vi "SaveVIlocations.vi"(10 "NamesAndLocnsArray":T1[](array[typedef]), 11 "configuration file path":path) -> ()   [LabVIEW 2020]
uses:
  <vilib>/Utility/miscctls.llb/LVRectTypeDef.ctl
  <vilib>/Utility/config.llb/Write Key (I32).vi
  <vilib>/Utility/config.llb/NI_LVConfig.lvlib
  <vilib>/Utility/config.llb/Write Key (Path).vi
  Anemometry Sub Vis/Controls/VInameSizePath.ctl
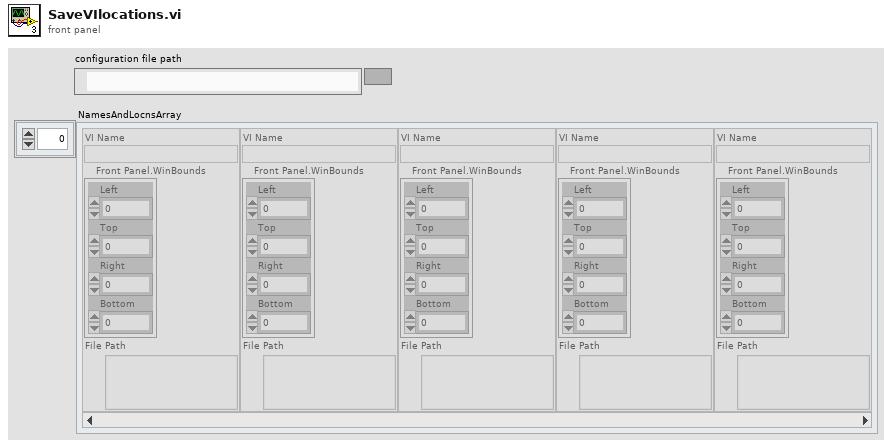
[diagram p1: front panel]
types:
  T1 = typedef "VInameSizePath.ctl" = cluster{"VI Name":string, "Front Panel.WinBounds":T2, "File Path":path}
  T2 = typedef "LVRectTypeDef.ctl" = cluster{"Left":i16, "Top":i16, "Right":i16, "Bottom":i16}
  T3 = typedef "NI_LVConfig.lvlib/Config Data RefNum.ctl" = refnum<k1>
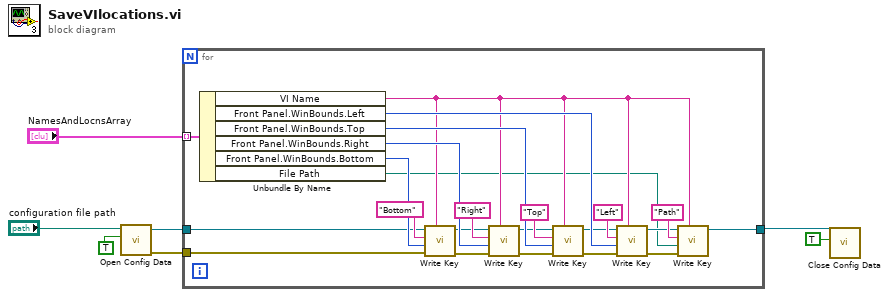
[diagram p0: block diagram]
diagram:
  n1 = call <vilib>:"Open Config Data.vi"("create file if necessary (T)"=TRUE, "configuration file path"="configuration file path") -> ("error out"=w3:errorcluster, "refnum"=w6:T3)  [unwired: 7 in, 1 out]
  n2 = for {
    tunnel: "NamesAndLocnsArray" -> [w30] mode=indexing
    tunnel: w6 -> [w18]
    tunnel: [w10] -> w5
    tunnel: w3 -> [w14]
    n3 = Unbundle By Name(w30) -> ("VI Name"=w9:string, "Front Panel.WinBounds.Left"=w26:i16, "Front Panel.WinBounds.Top"=w27:i16, "Front Panel.WinBounds.Right"=w28:i16, "Front Panel.WinBounds.Bottom"=w29:i16, "File Path"=w8:path)
    n4 = call-poly <vilib>:"Write Key.vi"("section"=w9, "error in (no error)"=w14, "value"=w29, "key"="Bottom", "refnum"=w18) -> ("error out"=w25:errorcluster, "refnum out"=w17:T3)  [unwired: 4 in, 1 out]
    n5 = call-poly <vilib>:"Write Key.vi"("section"=w9, "error in (no error)"=w25, "value"=w28, "key"="Right", "refnum"=w17) -> ("error out"=w24:errorcluster, "refnum out"=w16:T3)  [unwired: 4 in, 1 out]
    n6 = call-poly <vilib>:"Write Key.vi"("section"=w9, "error in (no error)"=w24, "value"=w27, "key"="Top", "refnum"=w16) -> ("error out"=w23:errorcluster, "refnum out"=w15:T3)  [unwired: 4 in, 1 out]
    n7 = call-poly <vilib>:"Write Key.vi"("section"=w9, "error in (no error)"=w23, "value"=w26, "key"="Left", "refnum"=w15) -> ("error out"=w12:errorcluster, "refnum out"=w11:T3)  [unwired: 4 in, 1 out]
    n8 = call-poly <vilib>:"Write Key.vi"("section"=w9, "error in (no error)"=w12, "value"=w8, "key"="Path", "refnum"=w11) -> ("refnum out"=w10:T3)  [unwired: 4 in, 2 out]
  }
  n9 = call <vilib>:"Close Config Data.vi"("write file if changed (T)"=TRUE, "refnum"=w5) -> ()  [unwired: 8 in, 2 out]
